vi "main_fg_usable_version.vi"() -> ()   [LabVIEW 2015]
uses:
  <vilib>/Instr/_visa.llb/VISA Configure Serial Port (Instr).vi
panel:
  out "Is conection open?":bool=TRUE
  in  "Boolean in":refnum<vi>
  in  "Attenuation":string(combo)
  in  "Level":dbl
  in  "Cmos":string(combo)
  in  "Duty":dbl=0.2 min=0.2 max=0.8 step=0.01
  in  "Modulation":string(combo)
  in  "Frequency":dbl=0.0001 min=0.0 max=0.5 step=0.001
  in  "Range":string(combo)
  in  "Offset":dbl min=-10.0 max=10.0 step=0.0001
  in  "Counter":string(combo)
  out "error out":errorcluster
  in  "Function type":string(combo)
  in  "close":bool=TRUE
  out "VISA resource name out":refnum<visa-resource-name>
  in  "open":bool=TRUE
  in  "VISA resource name":refnum<visa-resource-name>
  # "Initialize"
  # "Input/ output and error control"
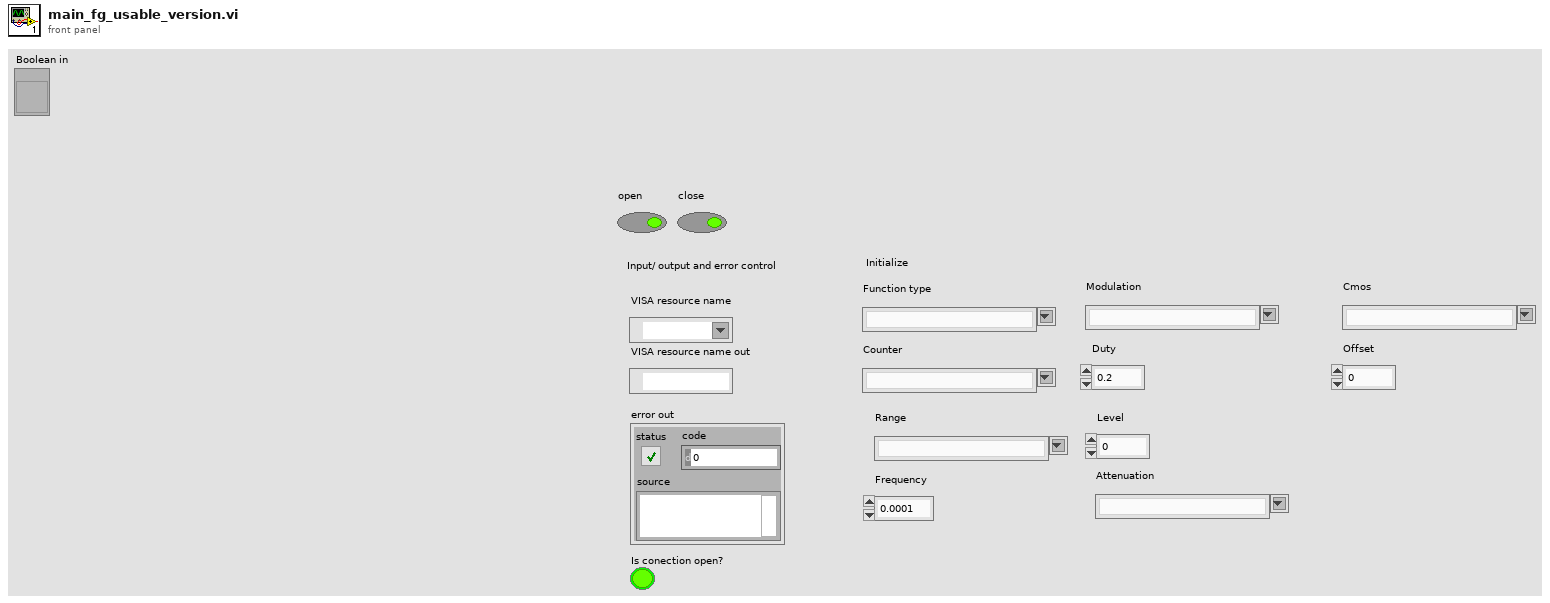
[diagram p1: front panel]
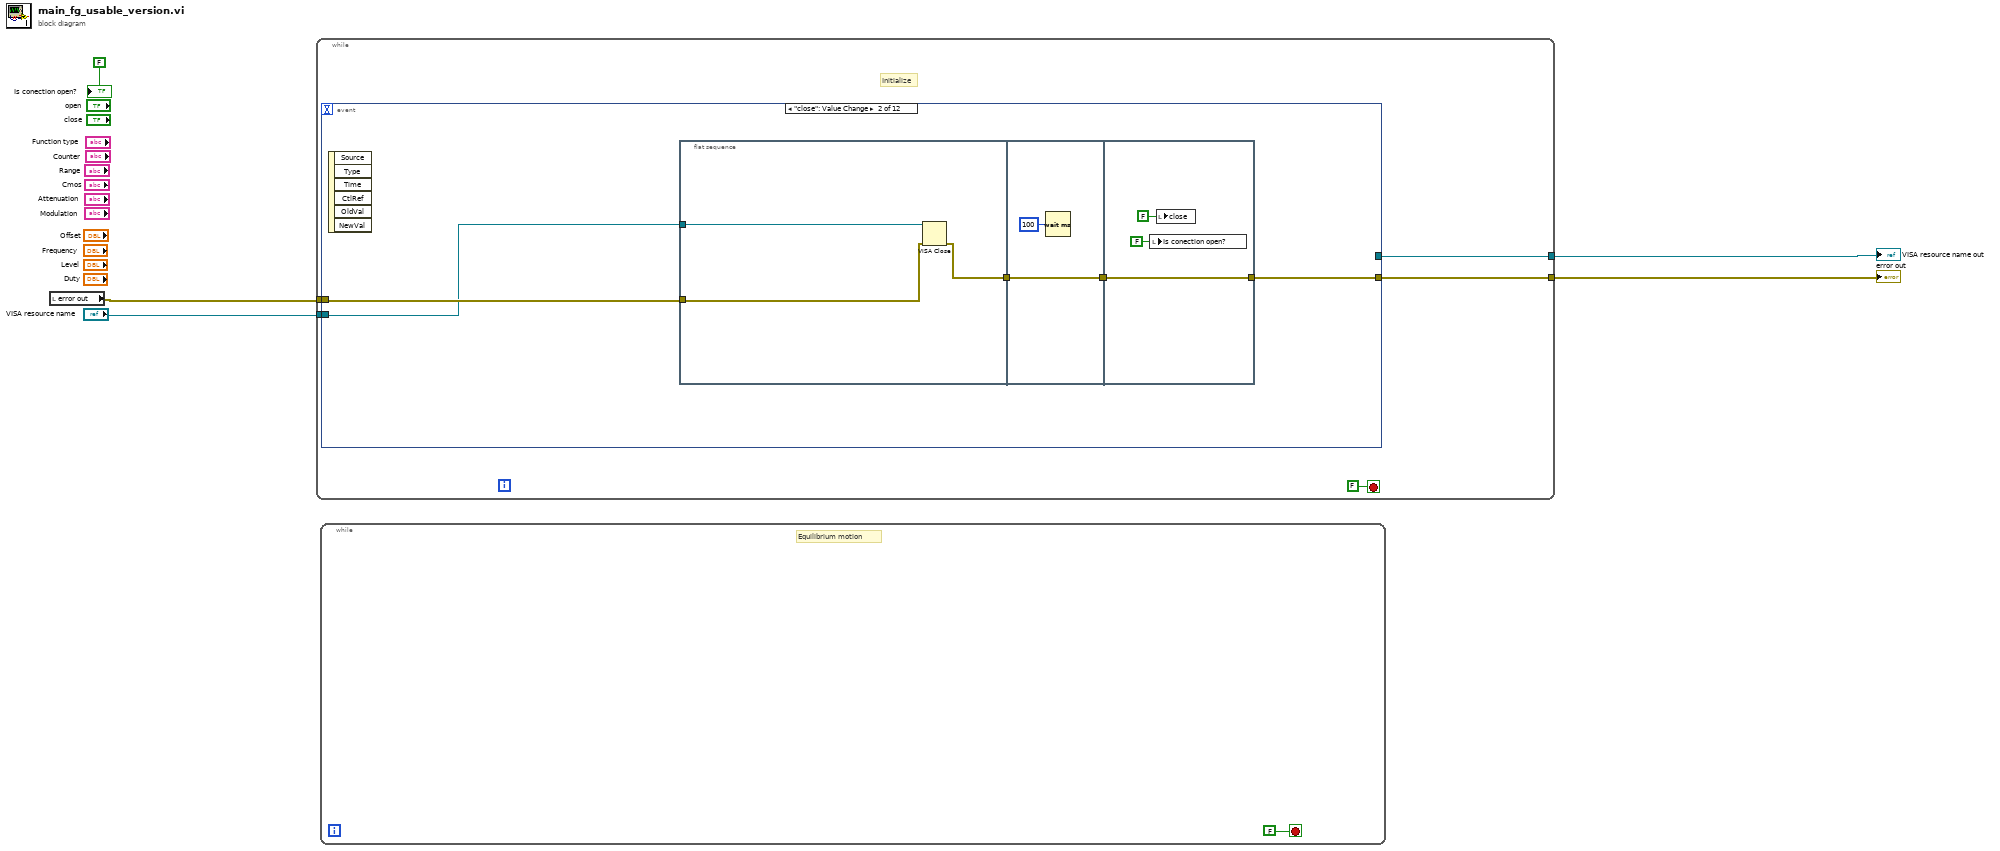
[diagram p0: block diagram]
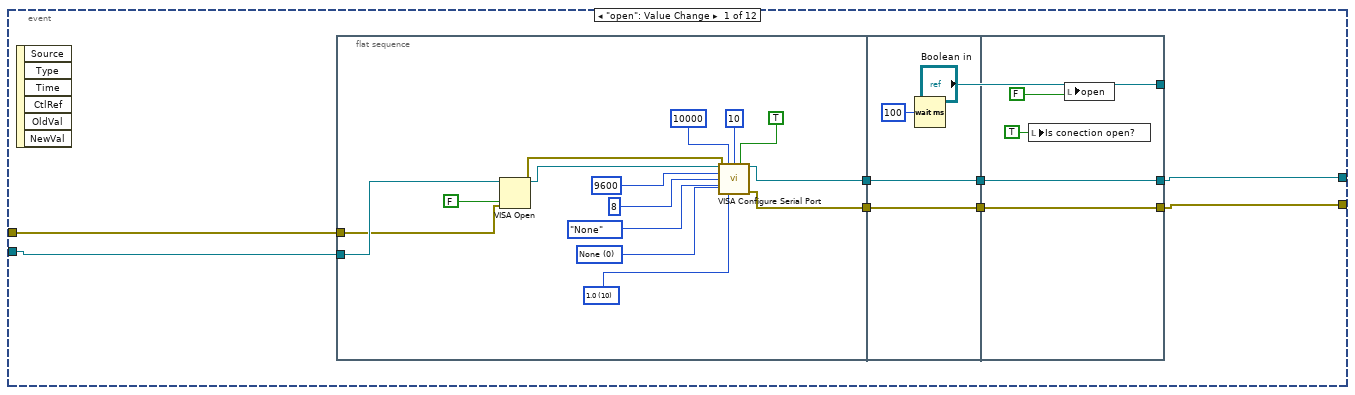
[diagram p2: hidden frame]
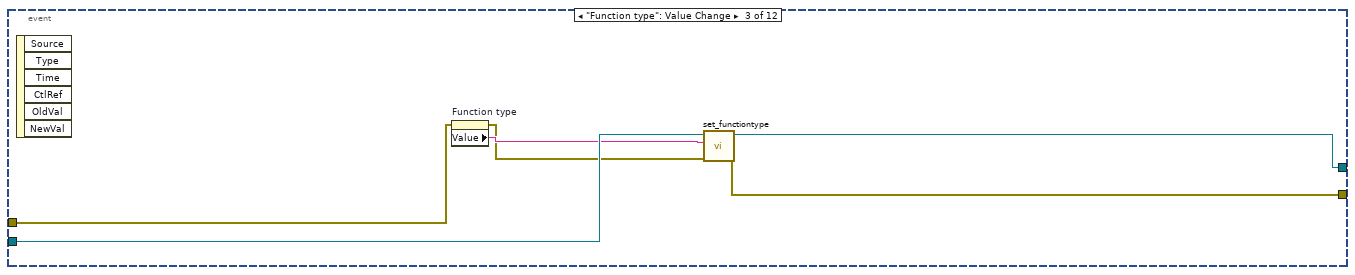
[diagram p3: hidden frame]
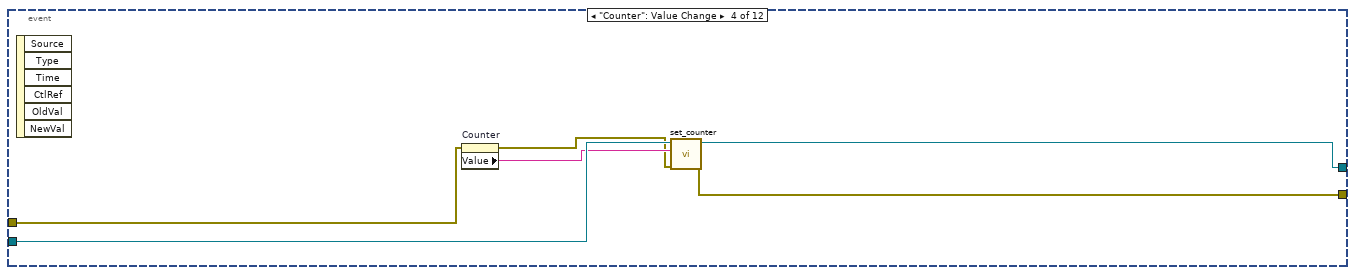
[diagram p4: hidden frame]
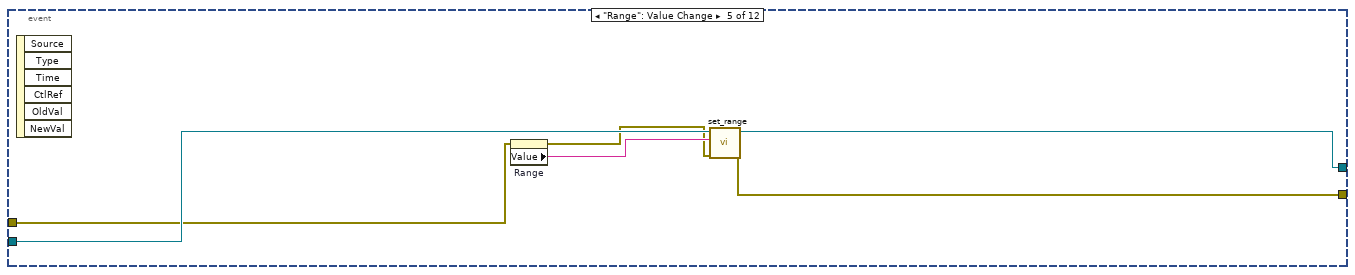
[diagram p5: hidden frame]
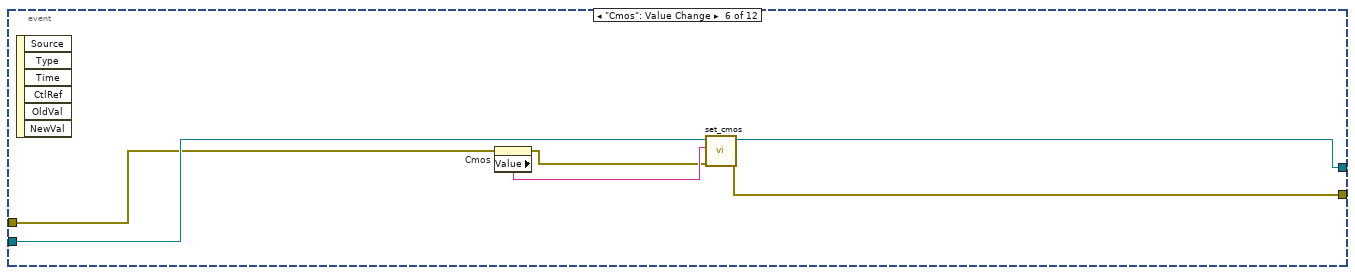
[diagram p6: hidden frame]
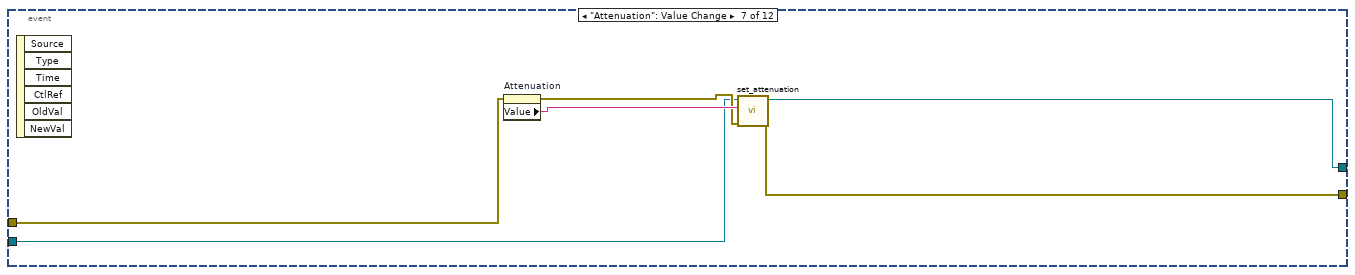
[diagram p7: hidden frame]
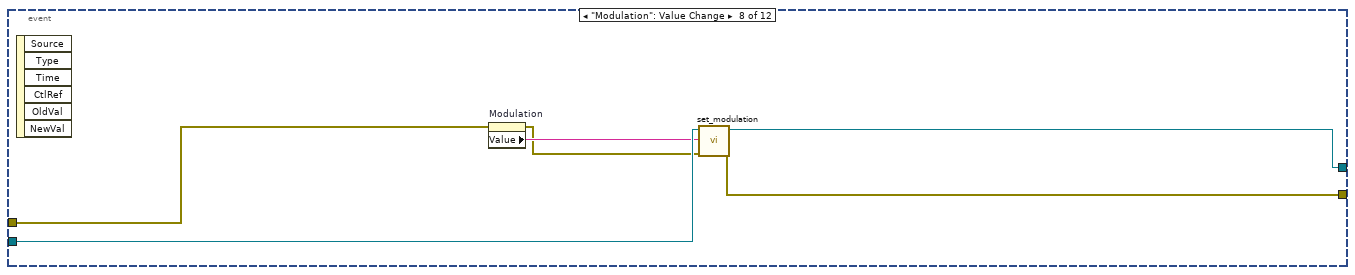
[diagram p8: hidden frame]
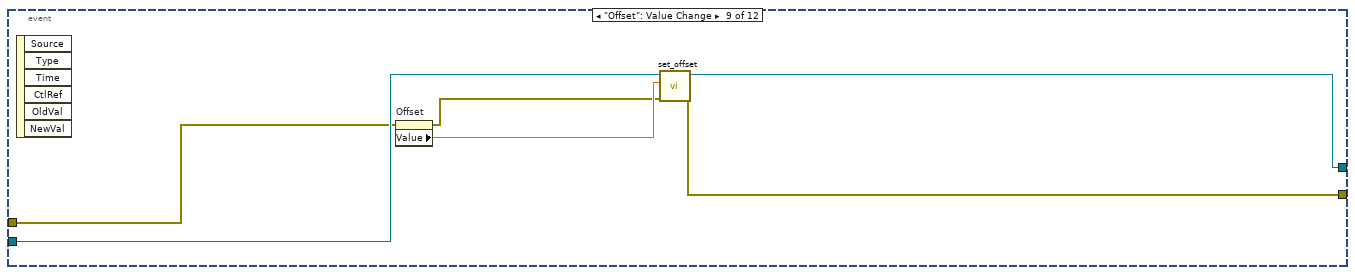
[diagram p9: hidden frame]
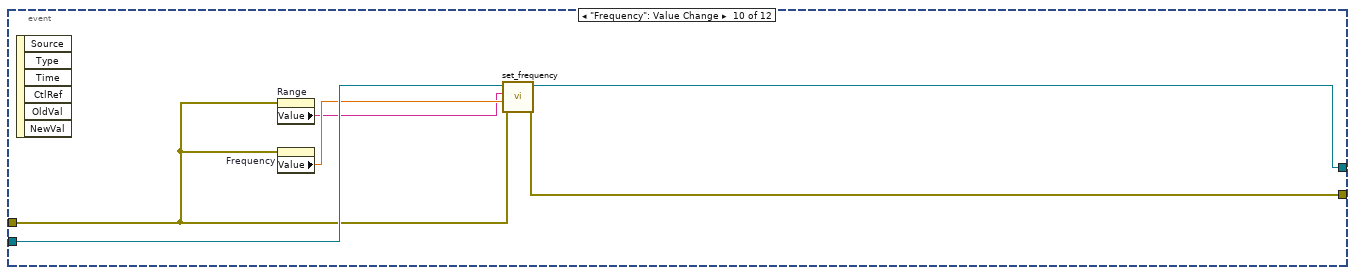
[diagram p10: hidden frame]
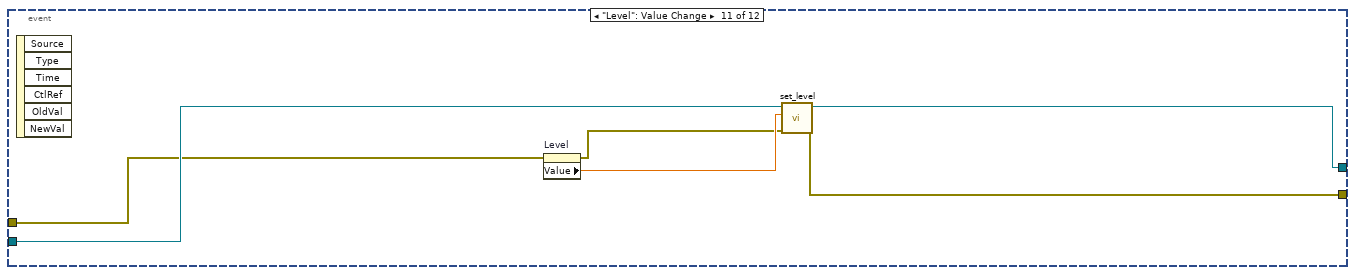
[diagram p11: hidden frame]
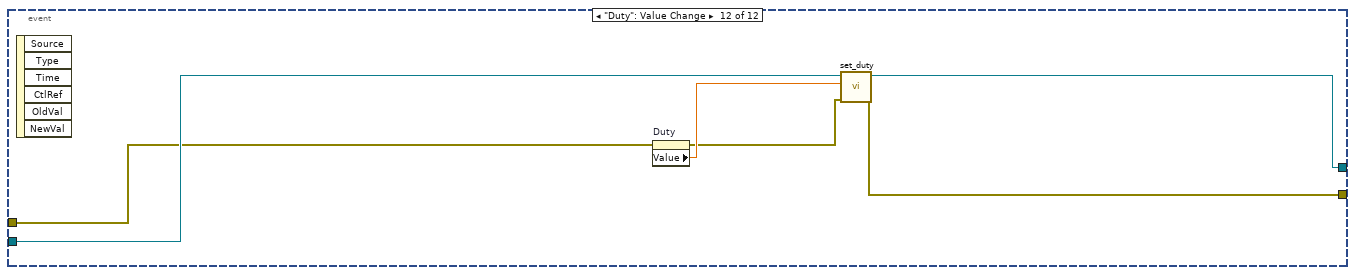
[diagram p12: hidden frame]
diagram:
  n1 = local read "error out"() -> (w5:errorcluster)
  n2 = while {
    tunnel: w5 -> [w8]
    tunnel: [w6] -> w4
    tunnel: "VISA resource name" -> [w9]
    tunnel: [w7] -> w2
    stop <- FALSE ("stop") stop-if-true
    # "Initialize"
    n3 = event shown="[1] \"close\": Value Change" {
      selector: _ -> [_ _ _ _ _ _ _ _ _ _ _ _]
      dyn-events: _ -> [_ _ _ _ _ _ _ _ _ _ _ _]
      timeout: _ -> [_ _ _ _ _ _ _ _ _ _ _ _]
      tunnel: w9 -> [w14 w44 w59 w64 w72 w78 w79 w90 w95 w102 w108 w114]
      tunnel: w8 -> [w13 w46 w56 w62 w68 w74 w80 w86 w92 w97 w104 w110]
      tunnel: [w12 _ w58 w65 w71 w76 w83 w89 w94 w101 w106 w113] -> w7
      tunnel: [w11 w45 w60 w66 w70 w77 w84 w88 w96 w100 w107 w112] -> w6
      event "open": Value Change {
        n4 = event-data() -> ()  [unwired: 1 in, 6 out]
        n5 = flat-sequence {
          tunnel: w14 -> [w33]
          tunnel: [w31] -> w19
          tunnel: [w30] -> w18
          tunnel: w13 -> [w20]
          tunnel: w19 -> [w37]
          tunnel: w18 -> [w36]
          tunnel: [w37] -> w17
          tunnel: [w36] -> w16
          tunnel: [w40] -> w11
          tunnel: [w41] -> w12
          tunnel: w17 -> [w41]
          tunnel: w16 -> [w40]
          tunnel: "Boolean in" -> [_]
          frame #0 {
            w21 = u16 0 items=["None", "XON/XOFF", "RTS/CTS", "XON/XOFF & RTS/CTS", "DTR/DSR", "XON/XOFF & DTR/DSR"] ("flow control (0:none)")
            w22 = u16 10 items=["1.0"=10, "1.5"=15, "2.0"=20] ("stop bits (10: 1 bit)")
            n6 = VISA Open(duplicate session (F)=FALSE, error in (no error)=w20, VISA resource name=w33) -> (VISA resource name=w32:refnum<visa-resource-name>, error out=w29:errorcluster)  [unwired: 2 in]
            n7 = call-poly "VISA Configure Serial Port"("VISA resource name"=w32, "timeout (10sec)"=u32 10000, "termination char\n(0xA = '\\n' = LF)"=u8 10 ("termination char\n(0xA = '\\n' = LF)"), "Enable Termination\nChar (T)"=TRUE ("Enable Termination\nChar (T)"), "baud rate (9600)"=u32 9600, "data bits (8)"=u16 8, "parity (0:none)"=enum16{"None", "Odd", "Even", "Mark", "Space"}."None", "error in (no error)"=w29, "stop bits (10: 1 bit)"=w22, "flow control (0:none)"=w21) -> ("VISA resource name out"=w31:refnum<visa-resource-name>, "error out"=w30:errorcluster)  [unwired: 4 in]
          }
          frame #1 {
            n8 = Wait (ms)(milliseconds to wait=u32 100) -> ()  [unwired: 1 out]
          }
          frame #2 {
            n9 = local write "Is conection open?"(TRUE ("Is conection open?")) -> ()
            n10 = local write "open"(FALSE) -> ()
          }
        }
      }
      event "close": Value Change {
        n11 = event-data() -> ()  [unwired: 1 in, 6 out]
        n12 = flat-sequence {
          tunnel: w46 -> [w49]
          tunnel: w44 -> [w47]
          tunnel: [w48] -> w43
          tunnel: w43 -> [w51]
          tunnel: [w51] -> w42
          tunnel: [w54] -> w45
          tunnel: w42 -> [w54]
          frame #0 {
            n13 = VISA Close(VISA resource name=w47, error in (no error)=w49) -> (error out=w48:errorcluster)
          }
          frame #1 {
            n14 = Wait (ms)(milliseconds to wait=u32 100) -> ()  [unwired: 1 out]
          }
          frame #2 {
            n15 = local write "Is conection open?"(FALSE ("Is conection open?")) -> ()
            n16 = local write "close"(FALSE ("close")) -> ()
          }
        }
      }
      event "Function type": Value Change {
        n17 = event-data() -> ()  [unwired: 1 in, 6 out]
        n18 = property on="Function type" class="CmbBox"(error in=w56) -> (error out=w55:errorcluster, "Value"=w57:string)  [unwired: 1 in, 1 out]
        n19 = call "set_functiontype.vi"("error in (no error)"=w55, "Value"=w57, "VISA Refnum in"=w59) -> ("error out"=w60:errorcluster, "VISA Refnum out"=w58:refnum<visa-resource-name>)  [unwired: 7 in]
      }
      event "Counter": Value Change {
        n20 = event-data() -> ()  [unwired: 1 in, 6 out]
        n21 = property on="Counter" class="CmbBox"(error in=w62) -> (error out=w61:errorcluster, "Value"=w63:string)  [unwired: 1 in, 1 out]
        n22 = call "set_counter.vi"("error in (no error)"=w61, "Value"=w63, "VISA Refnum in"=w64) -> ("error out"=w66:errorcluster, "VISA Refnum out"=w65:refnum<visa-resource-name>)  [unwired: 7 in]
      }
      event "Range": Value Change {
        n23 = event-data() -> ()  [unwired: 1 in, 6 out]
        n24 = property on="Range" class="CmbBox"(error in=w68) -> (error out=w67:errorcluster, "Value"=w69:string)  [unwired: 1 in, 1 out]
        n25 = call "set_range.vi"("error in (no error)"=w67, "Value"=w69, "VISA Refnum in"=w72) -> ("error out"=w70:errorcluster, "VISA Refnum out"=w71:refnum<visa-resource-name>)  [unwired: 7 in]
      }
      event "Cmos": Value Change {
        n26 = event-data() -> ()  [unwired: 1 in, 6 out]
        n27 = property on="Cmos" class="CmbBox"(error in=w74) -> (error out=w73:errorcluster, "Value"=w75:string)  [unwired: 1 in, 1 out]
        n28 = call "set_cmos.vi"("error in (no error)"=w73, "Value"=w75, "VISA Refnum in"=w78) -> ("error out"=w77:errorcluster, "VISA Refnum out"=w76:refnum<visa-resource-name>)  [unwired: 7 in]
      }
      event "Attenuation": Value Change {
        n29 = event-data() -> ()  [unwired: 1 in, 6 out]
        n30 = property on="Attenuation" class="CmbBox"(error in=w80) -> (error out=w81:errorcluster, "Value"=w82:string)  [unwired: 1 in, 1 out]
        n31 = call "set_attenuation.vi"("error in (no error)"=w81, "Value"=w82, "VISA Refnum in"=w79) -> ("error out"=w84:errorcluster, "VISA Refnum out"=w83:refnum<visa-resource-name>)  [unwired: 7 in]
      }
      event "Modulation": Value Change {
        n32 = event-data() -> ()  [unwired: 1 in, 6 out]
        n33 = property on="Modulation" class="CmbBox"(error in=w86) -> (error out=w85:errorcluster, "Value"=w87:string)  [unwired: 1 in, 1 out]
        n34 = call "set_modulation.vi"("error in (no error)"=w85, "Value"=w87, "VISA Refnum in"=w90) -> ("error out"=w88:errorcluster, "VISA Refnum out"=w89:refnum<visa-resource-name>)  [unwired: 7 in]
      }
      event "Offset": Value Change {
        n35 = event-data() -> ()  [unwired: 1 in, 6 out]
        n36 = property on="Offset" class="DigNum (strict)"(error in=w92) -> (error out=w91:errorcluster, "Value"=w93:dbl)  [unwired: 1 in, 1 out]
        n37 = call "set_offset.vi"("error in (no error)"=w91, "Value"=w93, "VISA Refnum in"=w95) -> ("error out"=w96:errorcluster, "VISA Refnum out"=w94:refnum<visa-resource-name>)  [unwired: 7 in]
      }
      event "Frequency": Value Change {
        n38 = event-data() -> ()  [unwired: 1 in, 6 out]
        n39 = property on="Range" class="CmbBox"(error in=w97) -> ("Value"=w98:string)  [unwired: 1 in, 2 out]
        n40 = property on="Frequency" class="DigNum (strict)"(error in=w97) -> ("Value"=w99:dbl)  [unwired: 1 in, 2 out]
        n41 = call "set_frequency.vi"("error in (no error)"=w97, "Value 2"=w99, "Value"=w98, "VISA Refnum in"=w102) -> ("error out"=w100:errorcluster, "VISA Refnum out"=w101:refnum<visa-resource-name>)  [unwired: 6 in]
      }
      event "Level": Value Change {
        n42 = event-data() -> ()  [unwired: 1 in, 6 out]
        n43 = property on="Level" class="DigNum (strict)"(error in=w104) -> (error out=w103:errorcluster, "Value"=w105:dbl)  [unwired: 1 in, 1 out]
        n44 = call "set_level.vi"("error in (no error)"=w103, "Value"=w105, "VISA Refnum in"=w108) -> ("error out"=w107:errorcluster, "VISA Refnum out"=w106:refnum<visa-resource-name>)  [unwired: 7 in]
      }
      event "Duty": Value Change {
        n45 = event-data() -> ()  [unwired: 1 in, 6 out]
        n46 = property on="Duty" class="DigNum (strict)"(error in=w110) -> (error out=w109:errorcluster, "Value"=w111:dbl)  [unwired: 1 in, 1 out]
        n47 = call "set_duty.vi"("error in (no error)"=w109, "Value"=w111, "VISA Refnum in"=w114) -> ("error out"=w112:errorcluster, "VISA Refnum out"=w113:refnum<visa-resource-name>)  [unwired: 7 in]
      }
    }
  }
  "error out" <- w4
  "VISA resource name out" <- w2
  n48 = while {
    stop <- FALSE stop-if-true
    # "Equilibrium motion"
  }
  "Is conection open?" <- FALSE ("Is conection open?")
